vi "read_matrix.vi"(8 "error in":errorcluster, 10 "Entry name":string, 11 "file refnum":refnum<file>) -> (0 "error out":errorcluster, 1 "Dimensions":i32[](array[numeric]), 2 "Result":dbl[][](array[numeric]), 3 "refnum out":refnum<file>, 4 "Found name":string)   [LabVIEW 2012]
panel:
  out "Type":string
  out "Lines":i32
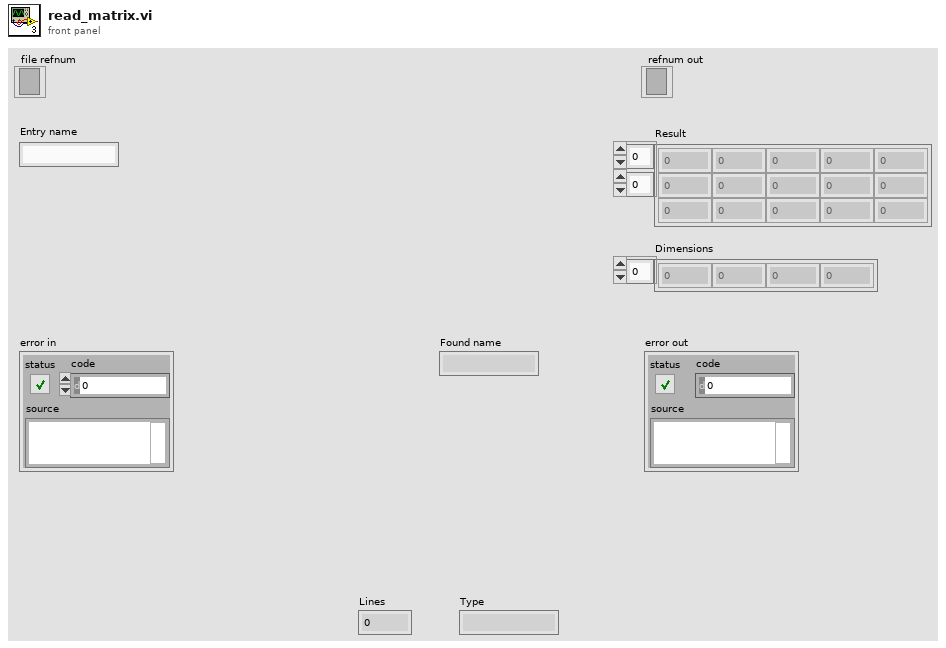
[diagram p1: front panel]
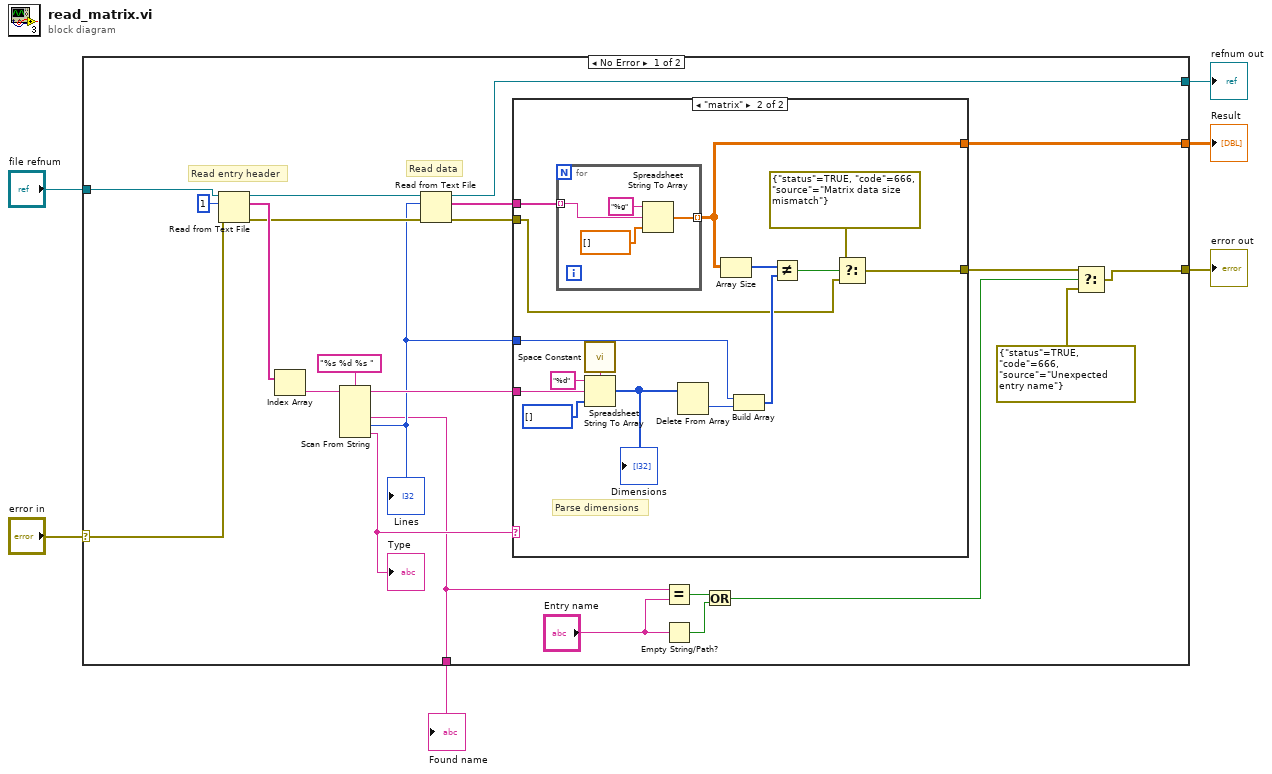
[diagram p0: block diagram]
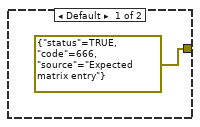
[diagram p2: hidden frame]
diagram:
  n1 = case shown="No Error" "error in" {
    selector: "error in" -> [w25 w50]
    tunnel: [w17 w51] -> w5
    tunnel: [w16 _] -> w4
    tunnel: [w8 w50] -> w3
    tunnel: [w15 _] -> w2
    tunnel: "file refnum" -> [w7 w51]
    frame No Error {
      # "Read data"
      # "Read entry header"
      n2 = Read from Text File(file (use dialog)=w7, count=1, error in=w25) -> (refnum out=w23:refnum<file>, text=w28:string[], error out=w24:errorcluster)  [unwired: 1 in, 1 out]
      n3 = Index Array(array=w28) -> (element=w27:string)  [unwired: 1 in]
      n4 = Scan From String(format string="%s %d %s ", input string=w27) -> (remaining string=w19:string, output 1=w15:string, output 2=w18:i32, output 3=w22:string)  [unwired: 5 in, 2 out]
      "Lines" <- w18
      "Type" <- w22
      n5 = Read from Text File(file (use dialog)=w23, count=w18, error in=w24) -> (refnum out=w17:refnum<file>, text=w20:string[], error out=w21:errorcluster)  [unwired: 1 in, 1 out]
      n6 = case shown="\"matrix\"" w22 {
        tunnel: w21 -> [_ w37]
        tunnel: w20 -> [_ w43]
        tunnel: w19 -> [_ w45]
        tunnel: w18 -> [_ w40]
        tunnel: [errorcluster {"status"=TRUE, "code"=666, "source"="Expected matrix entry"} ("t") w35] -> w11
        tunnel: [_ w34] -> w16
        frame Default {
        }
        frame "matrix" {
          # "Parse dimensions"
          n7 = for {
            tunnel: w43 -> [w48] mode=indexing
            tunnel: [w47] -> w34 mode=indexing
            n8 = Spreadsheet String To Array(format string="%g", spreadsheet string=w48, array type (2D Dbl)=dbl[] []) -> (array=w47:dbl[])  [unwired: 1 in]
          }
          n9 = call <vilib>:"Space Constant.vi"() -> ("String"=w42:string)
          n10 = Spreadsheet String To Array(delimiter (Tab)=w42, format string="%d", spreadsheet string=w45, array type (2D Dbl)=i32[] []) -> (array=w32:i32[])
          "Dimensions" <- w32
          n11 = Delete From Array(array=w32) -> (deleted portion=w31:i32)  [unwired: 2 in, 1 out]
          n12 = Array Size(array=w34) -> (size(s)=w41:i32[])
          n13 = Build Array(w40, w31) -> (w39:i32[])
          n14 = Not Equal?(x=w41, y=w39) -> (x != y?=w38:bool)
          n15 = Select(t=errorcluster {"status"=TRUE, "code"=666, "source"="Matrix data size mismatch"}, s=w38, f=w37) -> (s? t:f=w35:errorcluster)
        }
      }
      n16 = Equal?(x=w15, y="Entry name") -> (x = y?=w13:bool)
      n17 = Empty String/Path?(string/path="Entry name") -> (empty?=w12:bool)
      n18 = Or(x=w13, y=w12) -> (x .or. y?=w10:bool)
      n19 = Select(t=w11, s=w10, f=errorcluster {"status"=TRUE, "code"=666, "source"="Unexpected entry name"} ("t")) -> (s? t:f=w8:errorcluster)
    }
    frame Error {
    }
  }
  "refnum out" <- w5
  "Result" <- w4
  "error out" <- w3
  "Found name" <- w2
